vi "readUnicodeFile.vi"(8 "error in (no error)":errorcluster, 11 "Unicode File Path":path) -> (0 "error out":errorcluster, 3 "ASCII String":string)   [LabVIEW 2017, in "JKI Simple Localization.lvlib"]
uses:
  API/JKI Simple Localization.lvlib
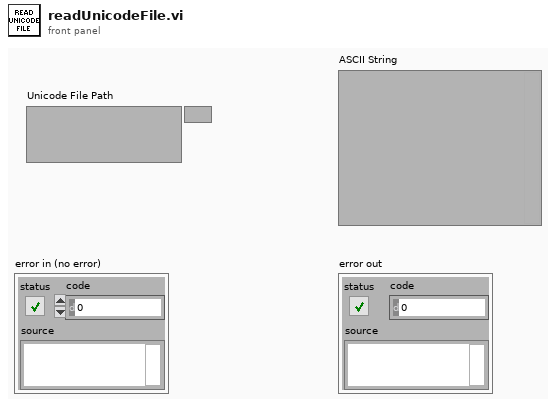
[diagram p1: front panel]
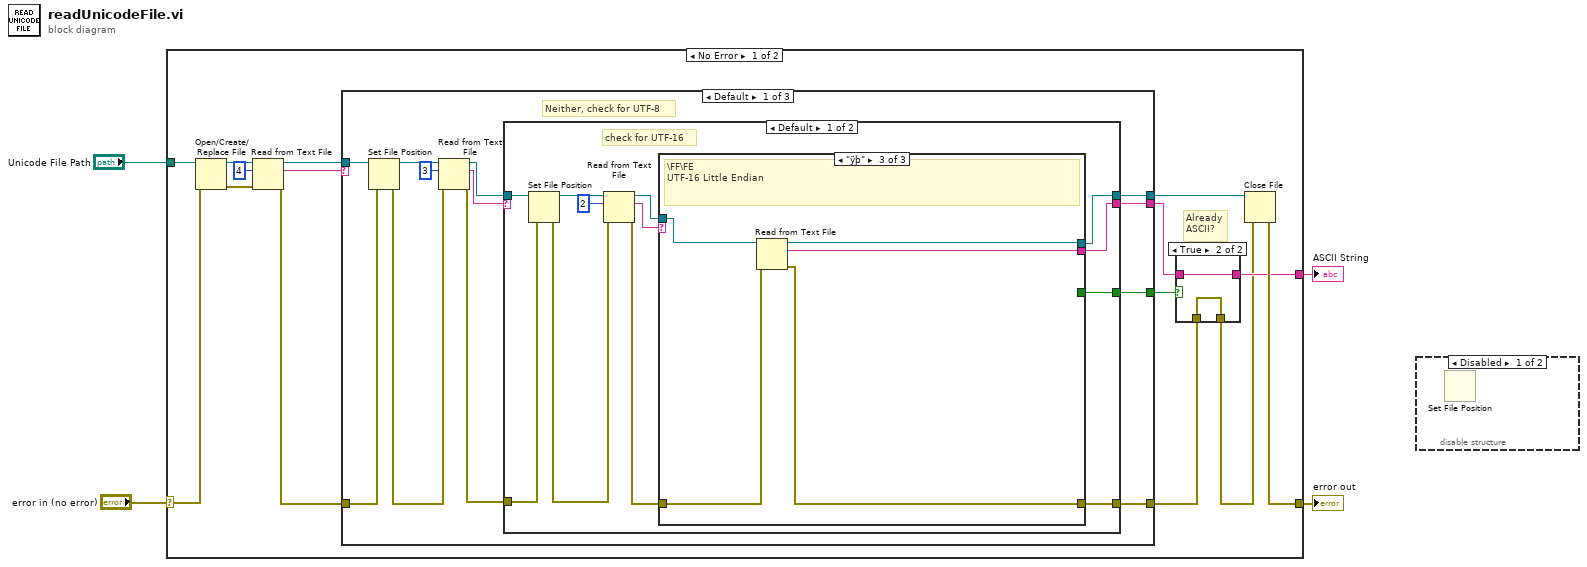
[diagram p0: block diagram]
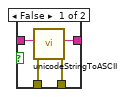
[diagram p2: hidden frame]
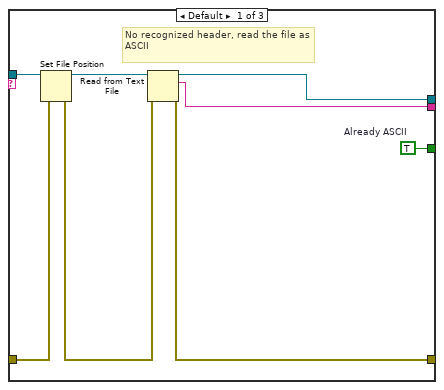
[diagram p3: hidden frame]
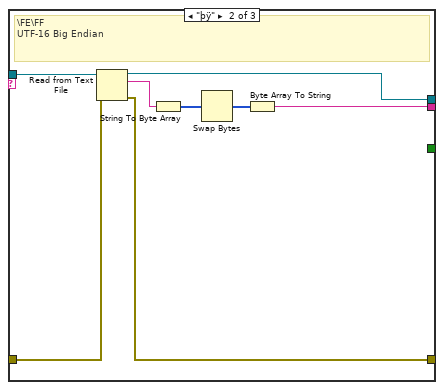
[diagram p4: hidden frame]
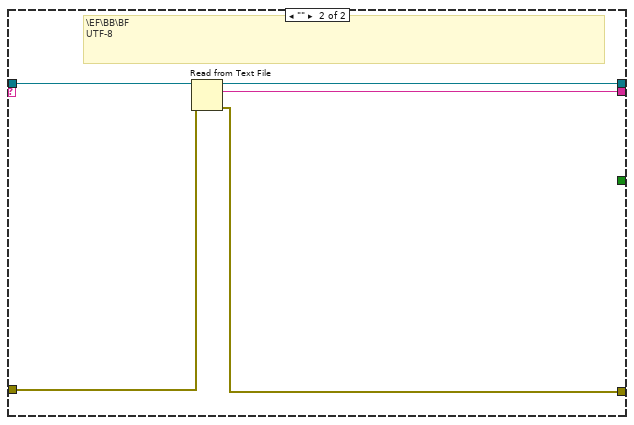
[diagram p5: hidden frame]
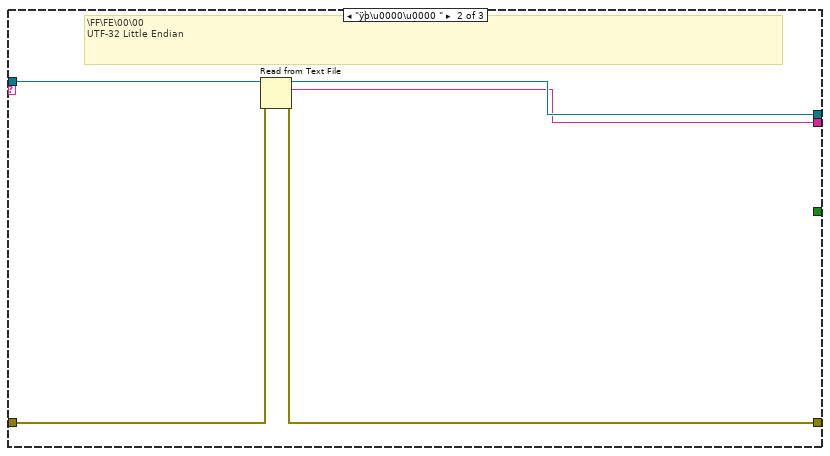
[diagram p6: hidden frame]
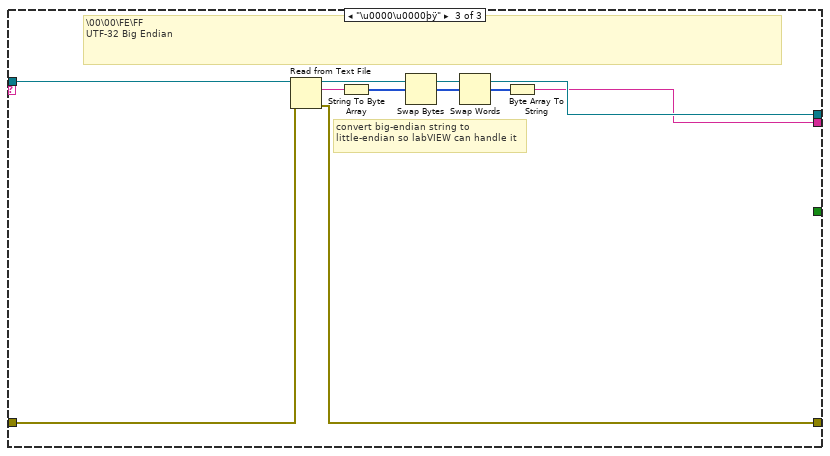
[diagram p7: hidden frame]
diagram:
  n1 = case shown="No Error" "error in (no error)" {
    selector: "error in (no error)" -> [w16 w90]
    tunnel: "Unicode File Path" -> [w19 _]
    tunnel: [w10 w90] -> w2
    tunnel: [w9 _] -> w1
    frame No Error {
      # "Already\nASCII?"
      n2 = Open/Create/Replace File(file path (use dialog)=w19, error in=w16) -> (refnum out=w18:refnum<file>, error out=w15:errorcluster)  [unwired: 4 in, 1 out]
      n3 = Read from Text File(file (use dialog)=w18, count=4, error in=w15) -> (refnum out=w13:refnum<file>, text=w14:string, error out=w12:errorcluster)  [unwired: 1 in, 1 out]
      n4 = case shown="Default" w14 {
        tunnel: w13 -> [w37 w80 w89]
        tunnel: w12 -> [w29 w79 w84]
        tunnel: [w32 w76 w81] -> w6
        tunnel: [w31 w77 w82] -> w8
        tunnel: [w27 w78 w83] -> w11
        tunnel: [w26 _ _] -> w7
        frame Default {
          # "Neither, check for UTF-8"
          n5 = Set File Position(refnum=w37, error in=w29) -> (refnum out=w30:refnum<file>, error out=w28:errorcluster)  [unwired: 2 in]
          n6 = Read from Text File(file (use dialog)=w30, count=3, error in=w28) -> (refnum out=w34:refnum<file>, text=w35:string, error out=w33:errorcluster)  [unwired: 1 in, 1 out]
          n7 = case shown="Default" w35 {
            tunnel: w34 -> [w49 w75]
            tunnel: w33 -> [w41 w74]
            tunnel: [w45 w72] -> w32
            tunnel: [w43 w71] -> w31
            tunnel: [w39 w73] -> w27
            tunnel: [w38 _] -> w26
            frame Default {
              # "check for UTF-16"
              n8 = Set File Position(refnum=w49, error in=w41) -> (refnum out=w42:refnum<file>, error out=w40:errorcluster)  [unwired: 2 in]
              n9 = Read from Text File(file (use dialog)=w42, count=2, error in=w40) -> (refnum out=w44:refnum<file>, text=w47:string, error out=w46:errorcluster)  [unwired: 1 in, 1 out]
              n10 = case shown="\"ÿþ\"" w47 {
                tunnel: w46 -> [w53 w61 w70]
                tunnel: [w55 w58 w66] -> w45
                tunnel: w44 -> [w57 w65 w68]
                tunnel: [w56 w59 w67] -> w43
                tunnel: [w51 w60 w69] -> w39
                tunnel: [w50 _ _] -> w38
                frame Default {
                  w50 = TRUE  # Already ASCII
                  # "No recognized header, read the file as ASCII"
                  n11 = Set File Position(refnum=w57, error in=w53) -> (refnum out=w54:refnum<file>, error out=w52:errorcluster)  [unwired: 2 in]
                  n12 = Read from Text File(file (use dialog)=w54, error in=w52) -> (refnum out=w51:refnum<file>, text=w56:string, error out=w55:errorcluster)  [unwired: 2 in, 1 out]
                }
                frame "þÿ" {
                  # "\\FE\\FF\nUTF-16 Big Endian"
                  n13 = Read from Text File(file (use dialog)=w65, error in=w61) -> (refnum out=w60:refnum<file>, text=w62:string, error out=w58:errorcluster)  [unwired: 2 in, 1 out]
                  n14 = String To Byte Array(string=w62) -> (unsigned byte array=w63:u8[])
                  n15 = Swap Bytes(anything=w63) -> (byte swapped=w64:u8[])
                  n16 = Byte Array To String(unsigned byte array=w64) -> (string=w59:string)
                }
                frame "ÿþ" {
                  # "\\FF\\FE\nUTF-16 Little Endian"
                  n17 = Read from Text File(file (use dialog)=w68, error in=w70) -> (refnum out=w69:refnum<file>, text=w67:string, error out=w66:errorcluster)  [unwired: 2 in, 1 out]
                }
              }
            }
            frame "﻿" {
              # "\\EF\\BB\\BF\nUTF-8"
              n18 = Read from Text File(file (use dialog)=w75, error in=w74) -> (refnum out=w73:refnum<file>, text=w71:string, error out=w72:errorcluster)  [unwired: 2 in, 1 out]
            }
          }
        }
        frame "ÿþ\u0000\u0000 " {
          # "\\FF\\FE\\00\\00\nUTF-32 Little Endian"
          n19 = Read from Text File(file (use dialog)=w80, error in=w79) -> (refnum out=w78:refnum<file>, text=w77:string, error out=w76:errorcluster)  [unwired: 2 in, 1 out]
        }
        frame "\u0000\u0000þÿ" {
          # "convert big-endian string to little-endian so labVIEW can handle it"
          # "\\00\\00\\FE\\FF \nUTF-32 Big Endian"
          n20 = Read from Text File(file (use dialog)=w89, error in=w84) -> (refnum out=w83:refnum<file>, text=w88:string, error out=w81:errorcluster)  [unwired: 2 in, 1 out]
          n21 = String To Byte Array(string=w88) -> (unsigned byte array=w86:u8[])
          n22 = Swap Bytes(anything=w86) -> (byte swapped=w87:u8[])
          n23 = Swap Words(1:w87) -> (0:w85:u8[])
          n24 = Byte Array To String(unsigned byte array=w85) -> (string=w82:string)
        }
      }
      n25 = case shown="True" w7 {
        tunnel: [w23 w25] -> w9
        tunnel: w8 -> [w22 w25]
        tunnel: w6 -> [w21 w24]
        tunnel: [w20 w24] -> w5
        frame False {
          n26 = call "unicodeStringToASCII.vi"("error in (no error)"=w21, "Unicode String"=w22) -> ("error out"=w20:errorcluster, "ASCII String"=w23:string)  [unwired: 8 in]
        }
        frame True {
        }
      }
      n27 = Close File(refnum=w11, error in=w5) -> (error out=w10:errorcluster)  [unwired: 1 out]
    }
    frame Error {
    }
  }
  "error out" <- w2
  "ASCII String" <- w1
  n28 = disable-structure shown="Disabled" {
    frame Disabled {
      n29 = Set File Position() -> ()  [unwired: 4 in, 2 out]
    }
    frame Enabled {
    }
  }
